vi "WS1050_51 VPI Header.vi"(8 "error in (no error)":errorcluster, 9 "WS1050/51":bool=TRUE, 10 "VPI_Cmd":string[](array[string])=["00", "3B", "00"], 11 "VPI Name":string[](array[string])=["All_Drivers OFF", "All Drivers ON", "All Drivers OFF2"]) -> (0 "error out":errorcluster, 1 "Cmd_3":string[](array[string]), 2 "VPI_3":string[](array[string]), 3 "VPI Header":string[](array[string]), 4 "Cmd_2":string[](array[string]), 5 "VPI_2":string[](array[string]), 6 "Cmd_1":string[](array[string]), 7 "VPI_1":string[](array[string]))   [LabVIEW 2012]
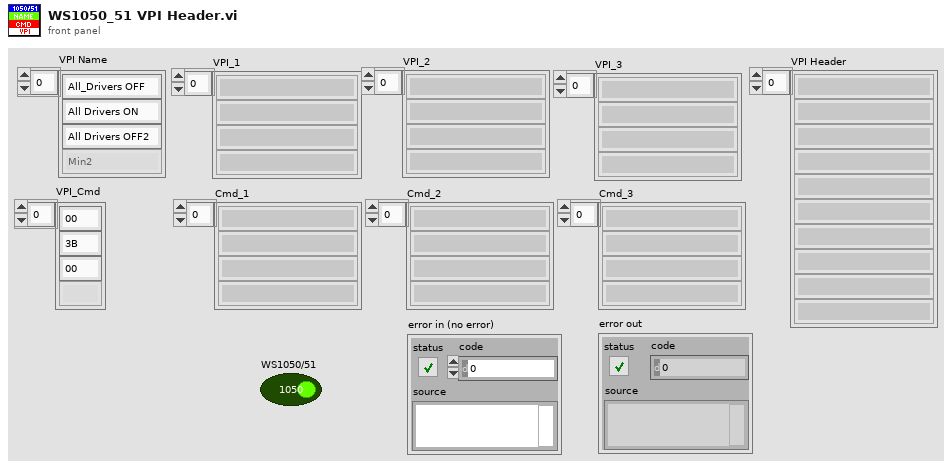
[diagram p1: front panel]
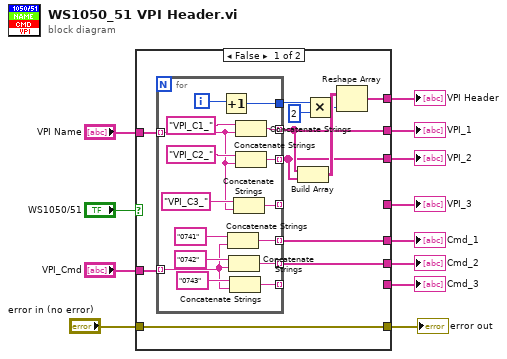
[diagram p0: block diagram]
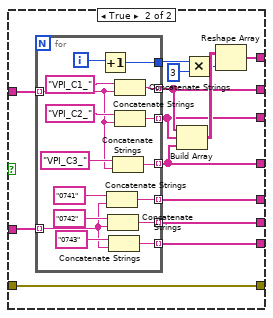
[diagram p2: hidden frame]
diagram:
  n1 = case shown="False" "WS1050/51" {
    tunnel: "error in (no error)" -> [w13 w50]
    tunnel: [w13 w50] -> w11
    tunnel: "VPI_Cmd" -> [w19 w49]
    tunnel: "VPI Name" -> [w20 w48]
    tunnel: [w18 w47] -> w7
    tunnel: [w17 w46] -> w6
    tunnel: [w16 w45] -> w5
    tunnel: [_ w44] -> w4
    tunnel: [w15 w43] -> w3
    tunnel: [w14 w42] -> w2
    tunnel: [_ w41] -> w1
    frame False {
      n2 = for {
        tunnel: w20 -> [w25] mode=indexing
        tunnel: w19 -> [w31] mode=indexing
        tunnel: [w37] -> w17 mode=indexing
        tunnel: [w36] -> w16 mode=indexing
        tunnel: [w35] -> _ mode=indexing
        tunnel: [w30] -> w15 mode=indexing
        tunnel: [w29] -> w14 mode=indexing
        tunnel: [w28] -> _ mode=indexing
        tunnel: [w26] -> w23
        i -> [w27]
        n3 = Increment(x=w27) -> (x+1=w26:i32)
        n4 = Concatenate Strings("0741" ("string"), w31) -> (w30:string)
        n5 = Concatenate Strings("0742" ("string"), w31) -> (w29:string)
        n6 = Concatenate Strings("0743" ("string"), w31) -> (w28:string)
        n7 = Concatenate Strings("VPI_C3_" ("string"), w25) -> (w35:string)
        n8 = Concatenate Strings("VPI_C1_" ("string"), w25) -> (w37:string)
        n9 = Concatenate Strings("VPI_C2_" ("string"), w25) -> (w36:string)
      }
      n10 = Build Array(w17, w16) -> (w24:string[][])
      n11 = Multiply(x=w23, y=2) -> (x*y=w22:i32)
      n12 = Reshape Array(w24, w22) -> (w18:string[])
    }
    frame True {
      n13 = for {
        tunnel: w48 -> [w55] mode=indexing
        tunnel: w49 -> [w61] mode=indexing
        tunnel: [w67] -> w46 mode=indexing
        tunnel: [w66] -> w45 mode=indexing
        tunnel: [w65] -> w44 mode=indexing
        tunnel: [w60] -> w43 mode=indexing
        tunnel: [w59] -> w42 mode=indexing
        tunnel: [w58] -> w41 mode=indexing
        tunnel: [w56] -> w53
        i -> [w57]
        n14 = Increment(x=w57) -> (x+1=w56:i32)
        n15 = Concatenate Strings("0741" ("string"), w61) -> (w60:string)
        n16 = Concatenate Strings("0742" ("string"), w61) -> (w59:string)
        n17 = Concatenate Strings("0743" ("string"), w61) -> (w58:string)
        n18 = Concatenate Strings("VPI_C3_" ("string"), w55) -> (w65:string)
        n19 = Concatenate Strings("VPI_C1_" ("string"), w55) -> (w67:string)
        n20 = Concatenate Strings("VPI_C2_" ("string"), w55) -> (w66:string)
      }
      n21 = Build Array(w46, w45, w44) -> (w54:string[][])
      n22 = Multiply(x=w53, y=3) -> (x*y=w52:i32)
      n23 = Reshape Array(w54, w52) -> (w47:string[])
    }
  }
  "error out" <- w11
  "VPI_1" <- w6
  "VPI_2" <- w5
  "VPI_3" <- w4
  "Cmd_1" <- w3
  "Cmd_2" <- w2
  "Cmd_3" <- w1
  "VPI Header" <- w7
